vi "MultiAnemo Receiver- hack.vi"() -> ()   [LabVIEW 2015]
doc: "Use this VI with the UDP Sender VI. Run this VI first.\n\nThe UDP protocol differs from TCP in that there is no error-checking with the packets of information that are sent, and thus no guarantee whatsoever that an intended recipient will actually receive a given piece of data.\n\nUDP does offer the ability to \"broadcast\" data across a network--simply specify an IP Address of all ones (255.255.255.255) to attempt to broadcast information network-wide. Keep in mind that routers and other network hardware will generally refuse to forward the broadcast beyond certain points, so the extent of the broadcast will in practice be limited."
uses:
  Anemometry/Anemometry Sub Vis/Globals/Meas_global.vi
panel:
  out "Numeric":i32
  in  "MOH3":u16=61563
  out "AnemoStringMOH3":string
  out "speedMOH3":dbl=nan
  in  "MOH2":u16=61562
  out "AnemoStringMOH2":string
  out "speedMOH2":dbl=nan
  in  "MOH1":u16=61561
  out "AnemoStringMOH1":string
  out "speedMOH1":dbl=nan
  out "Triggered":bool
  in  "Threshold":dbl=9.0
  out "speed2":dbl=nan
  out "speed1":dbl=nan
  out "AnemoString1":string
  in  "Veer1":u16=61557
  out "AnemoString2":string
  in  "max bytes/read":i32=548
  in  "Veer2":u16=61558
  in  "stop":bool
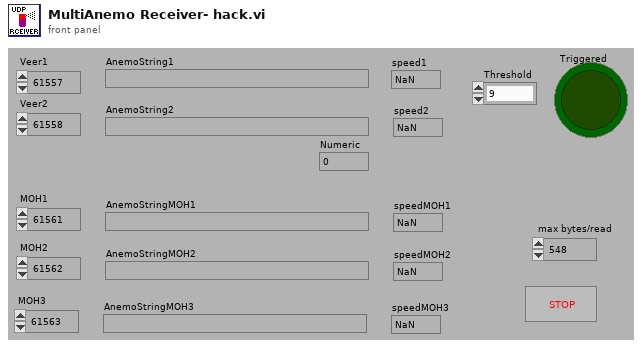
[diagram p1: front panel]
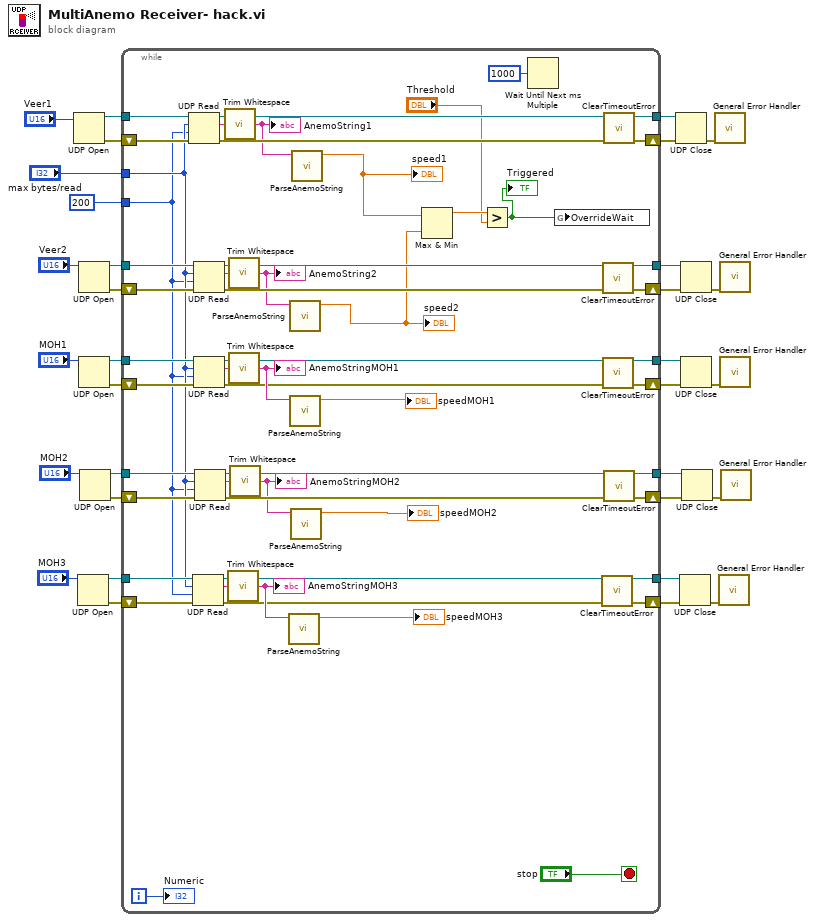
[diagram p0: block diagram]
diagram:
  n1 = UDP Open(11:"Veer1") -> (port=w21:refnum<k16>, 0:w20:errorcluster)  [unwired: 4 in, 1 out]
  n2 = UDP Open(11:"MOH3") -> (port=w3:refnum<k16>, 0:w2:errorcluster)  [unwired: 4 in, 1 out]
  n3 = UDP Open(11:"Veer2") -> (port=w30:refnum<k16>, 0:w31:errorcluster)  [unwired: 4 in, 1 out]
  n4 = UDP Open(11:"MOH1") -> (port=w15:refnum<k16>, 0:w14:errorcluster)  [unwired: 4 in, 1 out]
  n5 = UDP Open(11:"MOH2") -> (port=w10:refnum<k16>, 0:w11:errorcluster)  [unwired: 4 in, 1 out]
  n6 = while {
    tunnel: [w78] -> w29
    tunnel: w30 -> [w79]
    shift-left: w31 -> [w80]
    shift-right: [w76] -> w28
    tunnel: "max bytes/read" -> [w34]
    tunnel: 200 -> [w33]
    tunnel: [w71] -> w22
    tunnel: w21 -> [w70]
    shift-right: [w73] -> w23
    shift-left: w20 -> [w69]
    tunnel: [w56] -> w16
    tunnel: w15 -> [w55]
    shift-right: [w58] -> w17
    shift-left: w14 -> [w54]
    tunnel: [w51] -> w9
    tunnel: w10 -> [w52]
    shift-right: [w49] -> w8
    shift-left: w11 -> [w53]
    tunnel: [w42] -> w4
    tunnel: w3 -> [w41]
    shift-right: [w44] -> w5
    shift-left: w2 -> [w40]
    i -> [w35]
    stop <- "stop" stop-if-true
    n7 = UDP Read(connection ID=w70, max size (548)=w34, timeout ms (25000)=w33, 8:w69) -> (data out=w67:string, error out=w72:errorcluster, 3:w71:refnum<k16>)  [unwired: 2 out]
    n8 = UDP Read(connection ID=w41, max size (548)=w34, timeout ms (25000)=w33, 8:w40) -> (data out=w45:string, error out=w43:errorcluster, 3:w42:refnum<k16>)  [unwired: 2 out]
    n9 = UDP Read(connection ID=w79, max size (548)=w34, timeout ms (25000)=w33, 8:w80) -> (data out=w68:string, error out=w77:errorcluster, 3:w78:refnum<k16>)  [unwired: 2 out]
    n10 = UDP Read(connection ID=w55, max size (548)=w34, timeout ms (25000)=w33, 8:w54) -> (data out=w59:string, error out=w57:errorcluster, 3:w56:refnum<k16>)  [unwired: 2 out]
    n11 = UDP Read(connection ID=w52, max size (548)=w34, timeout ms (25000)=w33, 8:w53) -> (data out=w48:string, error out=w50:errorcluster, 3:w51:refnum<k16>)  [unwired: 2 out]
    n12 = call <vilib>:"Trim Whitespace.vi"("string"=w67) -> ("trimmed string"=w63:string)  [unwired: 1 in]
    "AnemoString1" <- w63
    n13 = call <vilib>:"Trim Whitespace.vi"("string"=w45) -> ("trimmed string"=w46:string)  [unwired: 1 in]
    "AnemoStringMOH3" <- w46
    n14 = call <vilib>:"Trim Whitespace.vi"("string"=w68) -> ("trimmed string"=w62:string)  [unwired: 1 in]
    "AnemoString2" <- w62
    n15 = call <vilib>:"Trim Whitespace.vi"("string"=w59) -> ("trimmed string"=w60:string)  [unwired: 1 in]
    "AnemoStringMOH1" <- w60
    n16 = call <vilib>:"Trim Whitespace.vi"("string"=w48) -> ("trimmed string"=w47:string)  [unwired: 1 in]
    "AnemoStringMOH2" <- w47
    n17 = call "ParseAnemoString.vi"("String"=w46) -> ("speed"=→"speedMOH3":dbl)  [unwired: 8 in, 2 out]
    n18 = call "ParseAnemoString.vi"("String"=w62) -> ("speed"=w39:dbl)  [unwired: 8 in, 2 out]
    "speed2" <- w39
    n19 = call "ParseAnemoString.vi"("String"=w60) -> ("speed"=→"speedMOH1":dbl)  [unwired: 8 in, 2 out]
    n20 = call "ParseAnemoString.vi"("String"=w47) -> ("speed"=→"speedMOH2":dbl)  [unwired: 8 in, 2 out]
    n21 = call "ParseAnemoString.vi"("String"=w63) -> ("speed"=w61:dbl)  [unwired: 8 in, 2 out]
    "speed1" <- w61
    n22 = Max & Min(x=w61, y=w39) -> (max(x,y)=w66:dbl)  [unwired: 1 out]
    n23 = Greater?(x=w66, y="Threshold") -> (0:w64:bool)
    "Triggered" <- w64
    n24 = Wait Until Next ms Multiple(millisecond multiple=u32 1000) -> ()  [unwired: 1 out]
    n25 = global write "Meas_global.vi" "OverrideWait"(w64) -> ()
    n26 = call "ClearTimeoutError.vi"("error in (no error)"=w43) -> ("error out"=w44:errorcluster)
    n27 = call "ClearTimeoutError.vi"("error in (no error)"=w77) -> ("error out"=w76:errorcluster)
    n28 = call "ClearTimeoutError.vi"("error in (no error)"=w57) -> ("error out"=w58:errorcluster)
    n29 = call "ClearTimeoutError.vi"("error in (no error)"=w72) -> ("error out"=w73:errorcluster)
    n30 = call "ClearTimeoutError.vi"("error in (no error)"=w50) -> ("error out"=w49:errorcluster)
    "Numeric" <- w35
  }
  n31 = UDP Close(connection ID=w22, 8:w23) -> (error out=w24:errorcluster)  [unwired: 1 out]
  n32 = UDP Close(connection ID=w4, 8:w5) -> (error out=w6:errorcluster)  [unwired: 1 out]
  n33 = UDP Close(connection ID=w29, 8:w28) -> (error out=w27:errorcluster)  [unwired: 1 out]
  n34 = UDP Close(connection ID=w16, 8:w17) -> (error out=w18:errorcluster)  [unwired: 1 out]
  n35 = UDP Close(connection ID=w9, 8:w8) -> (error out=w7:errorcluster)  [unwired: 1 out]
  n36 = call <vilib>:"General Error Handler.vi"("error in (no error)"=w24) -> ()  [unwired: 10 in, 5 out]
  n37 = call <vilib>:"General Error Handler.vi"("error in (no error)"=w6) -> ()  [unwired: 10 in, 5 out]
  n38 = call <vilib>:"General Error Handler.vi"("error in (no error)"=w27) -> ()  [unwired: 10 in, 5 out]
  n39 = call <vilib>:"General Error Handler.vi"("error in (no error)"=w18) -> ()  [unwired: 10 in, 5 out]
  n40 = call <vilib>:"General Error Handler.vi"("error in (no error)"=w7) -> ()  [unwired: 10 in, 5 out]
